vi "RCD TESTING.vi"(0 "Lock in Input":T1, 1 "error in (no error)":errorcluster, 2 "Deceleration":bool, 5 "RESET":bool, 6 "Accelaration":bool, 7 "B axis":i32, 8 "Stop":bool, 9 "A axis":i32, 10 "Comport":refnum<visa-resource-name>="COM4") -> (3 "A out":dbl, 4 "VISA resource name out":refnum<visa-resource-name>)   [LabVIEW 2020]
uses:
  <vilib>/Instr/_visa.llb/VISA Configure Serial Port (Instr).vi
  Dependencies/Holmarc/2 axis linear/GlobalValue.vi
  <vilib>/Utility/file.llb/Write Delimited Spreadsheet (DBL).vi
  Dependencies/Stanford Research 830/Stanford Research 830.lvlib
panel:
  out "Waveform Graph":sgl[](graph)
  in  "Maximum Time (10000 ms)":u32=10000
  in  "Continuous Storage (T: Enable)":bool=TRUE
  in  "Reset (True)":bool=TRUE
  in  "Sample Rate (0: 62.5 mHz)":u16(ring) items=["62.5 mHz", "125 mHz", "250 mHz", "500 mHz", "1 Hz", "2 Hz", "4 Hz", "8Hz", "16 Hz", "32 Hz", "64 Hz", "128 Hz", "256 Hz", "512 Hz", "Trigger "]
  out "error out 2":errorcluster
  out "B out":dbl
  # "COMPORT"
  # "To Move"
  # "Moved"
  # "Microns"
  # "Microns"
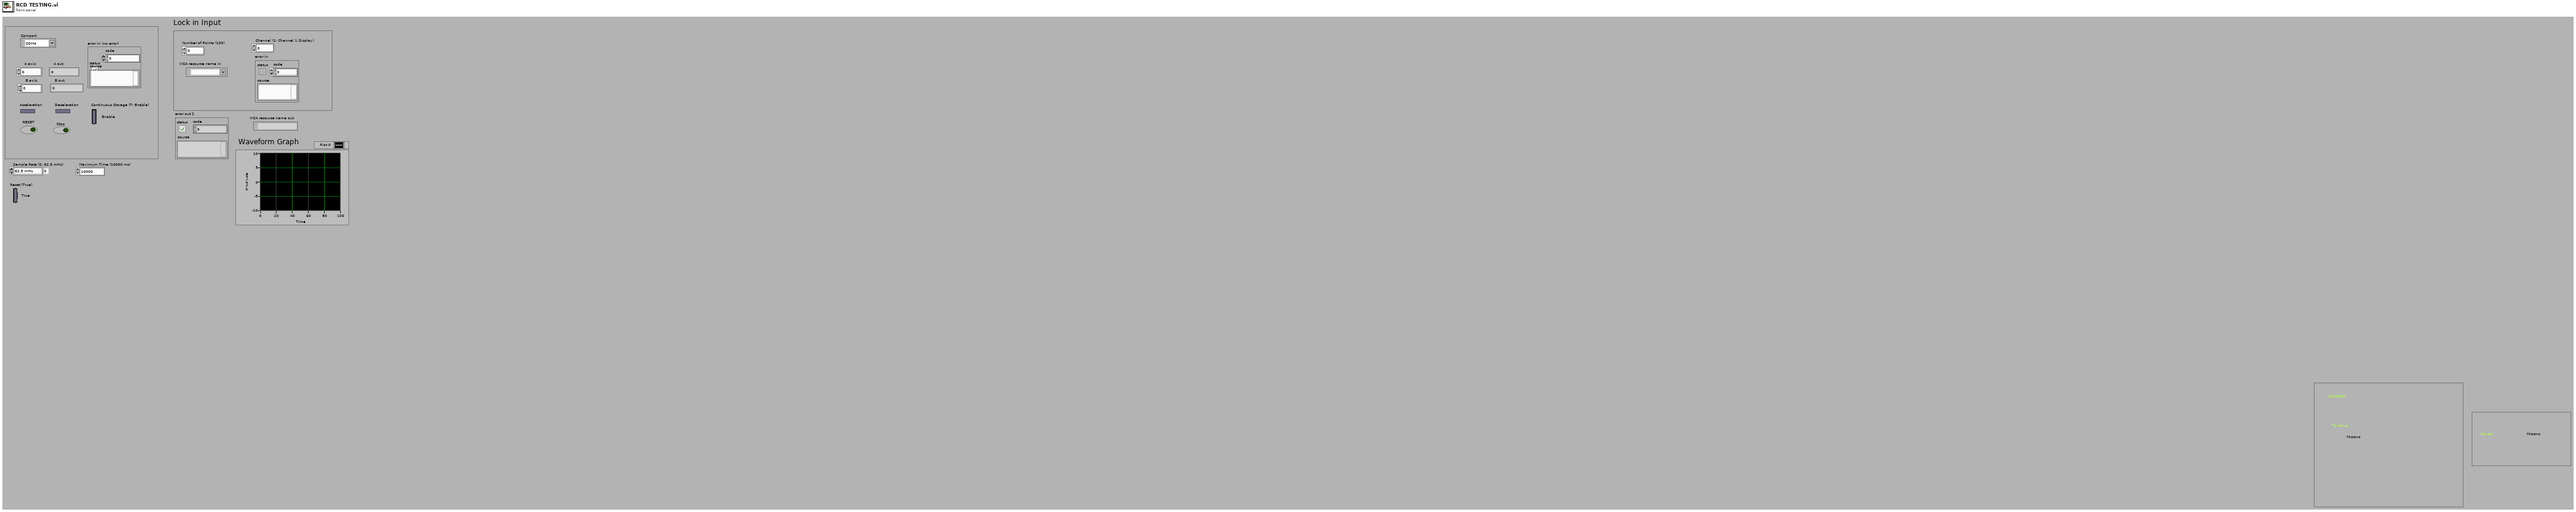
[diagram p1: front panel]
types:
  T1 = cluster{"Number of Points (100)":u32, "VISA resource name in":refnum<visa-resource-name>, "Channel (1: Channel 1 Display)":u16, "error in":errorcluster}
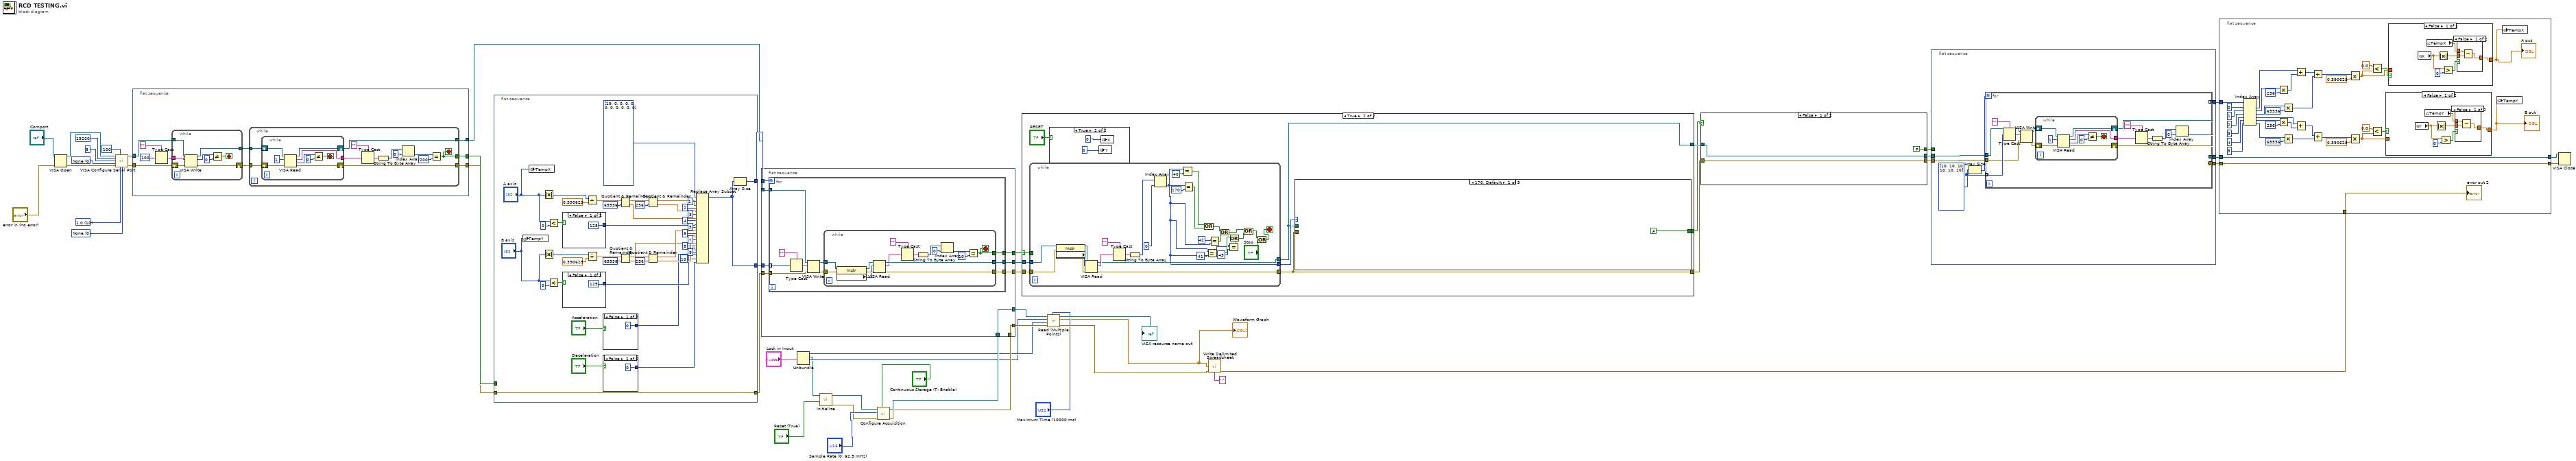
[diagram p0: block diagram]
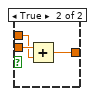
[diagram p2: hidden frame]
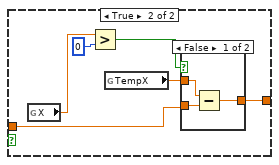
[diagram p3: hidden frame]
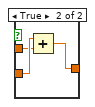
[diagram p4: hidden frame]
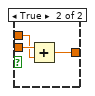
[diagram p5: hidden frame]
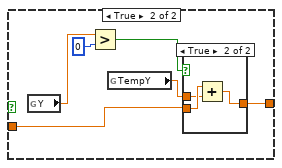
[diagram p6: hidden frame]
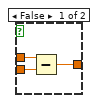
[diagram p7: hidden frame]
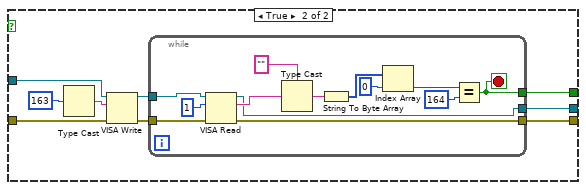
[diagram p8: hidden frame]
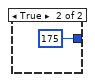
[diagram p9: hidden frame]
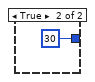
[diagram p10: hidden frame]
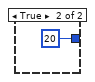
[diagram p11: hidden frame]
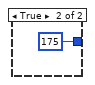
[diagram p12: hidden frame]
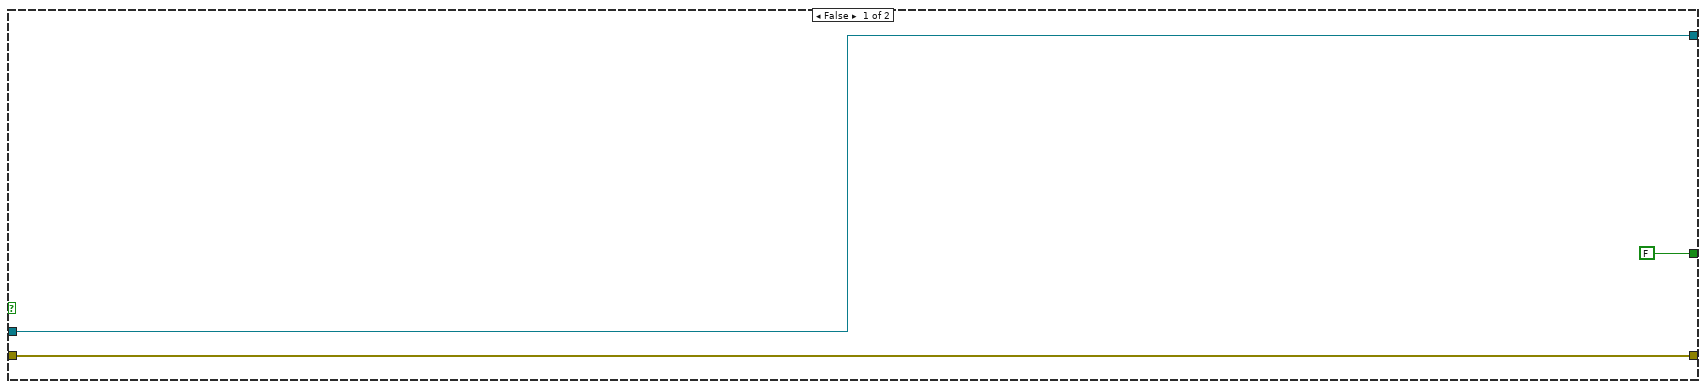
[diagram p13: hidden frame]
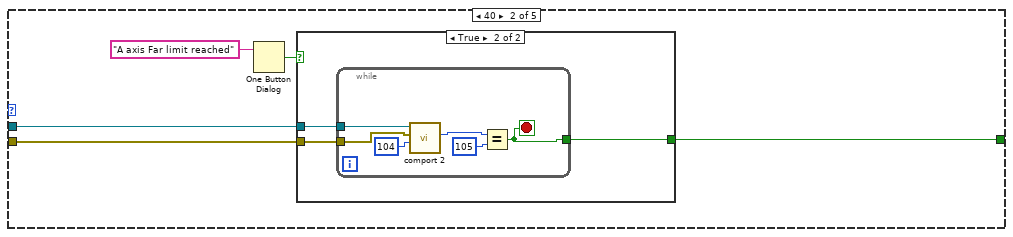
[diagram p15: hidden frame]
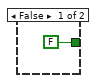
[diagram p16: hidden frame]
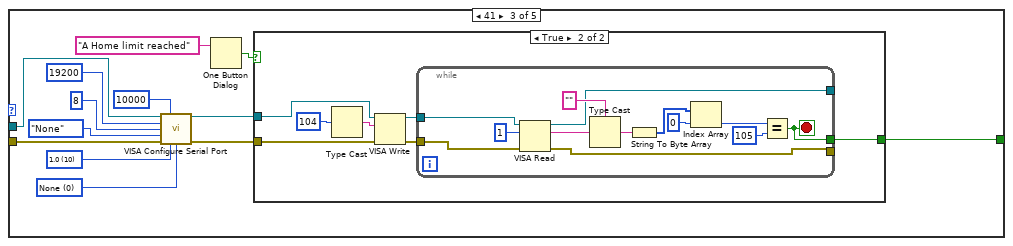
[diagram p17: hidden frame]
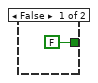
[diagram p18: hidden frame]
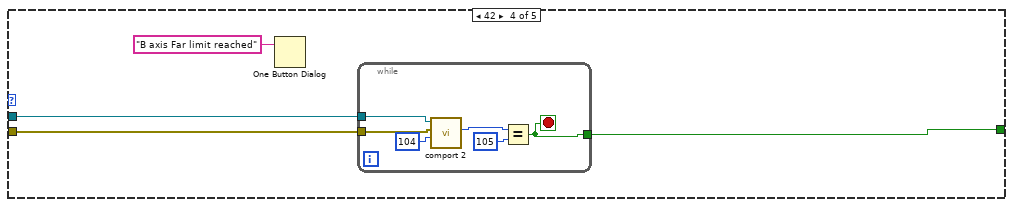
[diagram p19: hidden frame]
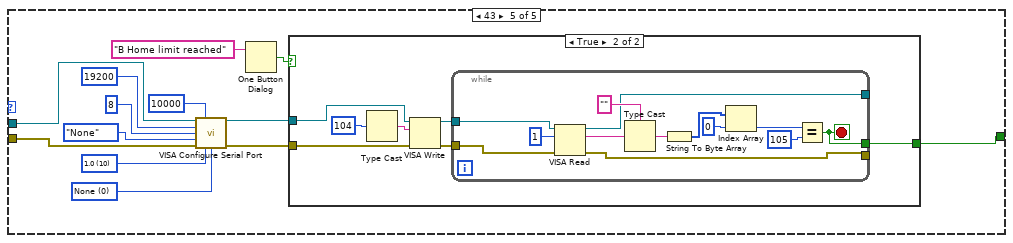
[diagram p20: hidden frame]
diagram:
  w46 = u16 0 items=["None"=0, "XON/XOFF"=1, "RTS/CTS"=2, "DTR/DSR"=4] ("flow control")
  w45 = u16 10 items=["1.0"=10, "1.5"=15, "2.0"=20] ("stop bits")
  w44 = u16 0 items=["None", "Odd", "Even", "Mark", "Space"] ("parity")
  n1 = VISA Open(error in (no error)="error in (no error)", VISA resource name="Comport") -> (VISA resource name=w49:refnum<visa-resource-name>, error out=w50:errorcluster)  [unwired: 3 in]
  n2 = call-poly "VISA Configure Serial Port"("VISA resource name"=w49, "timeout (10sec)"=u32 100, "baud rate (9600)"=u32 19200 ("baud rate"), "data bits (8)"=u16 8 ("data bits"), "parity (0:none)"=w44, "error in (no error)"=w50, "stop bits (10: 1 bit)"=w45, "flow control (0:none)"=w46) -> ("VISA resource name out"=w41:refnum<visa-resource-name>, "error out"=w40:errorcluster)  [unwired: 1 in, 5 out]
  n3 = flat-sequence {
    tunnel: w41 -> [w61]
    tunnel: w40 -> [w60]
    tunnel: [w59] -> w38
    tunnel: [w58] -> w25
    tunnel: [w52] -> w26
    frame #0 {
      n4 = Type Cast(type="", x=u8 100) -> (*(type *) &x=w56:string)
      n5 = while {
        tunnel: w56 -> [w69]
        shift-right: [w65] -> w53
        shift-left: w60 -> [w67]
        tunnel: w61 -> [w68]
        tunnel: [w66] -> w54
        stop <- w62 stop-if-true
        n6 = VISA Write(VISA resource name=w68, write buffer=w69, error in (no error)=w67) -> (VISA resource name out=w66:refnum<visa-resource-name>, return count=w64:u32, error out=w65:errorcluster)
        n7 = Not Equal?(x=w64, y=u32 0) -> (x != y?=w62:bool)
      }
      n8 = while {
        tunnel: w53 -> [w80]
        tunnel: [w78] -> w58
        tunnel: w54 -> [w81]
        tunnel: [w79] -> w59
        tunnel: [w73] -> w52
        stop <- w73 stop-if-true
        n9 = while {
          tunnel: [w85] -> w72
          shift-right: [w88] -> w79
          shift-left: w81 -> [w90]
          shift-right: [w87] -> w78
          shift-left: w80 -> [w89]
          stop <- w82 stop-if-true
          n10 = VISA Read(VISA resource name=w90, byte count=u32 1, error in (no error)=w89) -> (VISA resource name out=w88:refnum<visa-resource-name>, read buffer=w85:string, return count=w83:u32, error out=w87:errorcluster)
          n11 = Not Equal?(x=w83, y=u32 0) -> (x != y?=w82:bool)
        }
        n12 = Type Cast(type="", x=w72) -> (*(type *) &x=w70:string)
        n13 = String To Byte Array(string=w70) -> (unsigned byte array=w77:u8[])
        n14 = Index Array(array=w77, index=0) -> (element=w75:u8)
        n15 = Equal?(x=w75, y=u8 200) -> (x = y?=w73:bool)
      }
    }
  }
  n16 = flat-sequence {
    tunnel: [w129] -> w39
    tunnel: [w91] -> w37
    tunnel: w26 -> [_]
    tunnel: w25 -> [w126]
    tunnel: [w126] -> w24
    frame #0 {
      n17 = global write "GlobalValue.vi" "TempY"("B axis") -> ()
      n18 = global write "GlobalValue.vi" "TempX"("A axis") -> ()
      n19 = Absolute Value(x="A axis") -> (abs(x)=w130:i32)
      n20 = Absolute Value(x="B axis") -> (abs(x)=w118:i32)
      n21 = Less?(x="A axis", y=0) -> (x < y?=w132:bool)
      n22 = Less?(x="B axis", y=0) -> (x < y?=w113:bool)
      n23 = case shown="False" w132 {
        tunnel: [u16 125 u16 175] -> w104
        frame False {
        }
        frame True {
        }
      }
      n24 = case shown="False" w113 {
        tunnel: [u16 125 u16 175] -> w96
        frame False {
        }
        frame True {
        }
      }
      n25 = Divide(x=w130, y=0.390625) -> (x/y=w125:dbl)
      n26 = Divide(x=w118, y=0.390625) -> (x/y=w117:dbl)
      n27 = case shown="False" "Accelaration" {
        tunnel: [0 20] -> w94
        frame False {
        }
        frame True {
        }
      }
      n28 = case shown="False" "Deceleration" {
        tunnel: [0 30] -> w92
        frame False {
        }
        frame True {
        }
      }
      n29 = Quotient & Remainder(x=w125, y=65536) -> (x-y*floor(x/y)=w123:dbl, floor(x/y)=w107:dbl)
      n30 = Quotient & Remainder(x=w117, y=65536) -> (x-y*floor(x/y)=w115:dbl, floor(x/y)=w98:dbl)
      n31 = Quotient & Remainder(x=w123, y=256) -> (x-y*floor(x/y)=w110:dbl, floor(x/y)=w109:dbl)
      n32 = Quotient & Remainder(x=w115, y=256) -> (x-y*floor(x/y)=w102:dbl, floor(x/y)=w100:dbl)
      n33 = Replace Array Subset(array=u8[] [19, 0, 0, 0, 0, 0, 0, 0, 0, 0, 0], new element #1=w110, index #1=1 ("index"), new element #2=w109, index #2=2 ("index"), new element #3=w107, index #3=3 ("index"), new element #4=w104, index #4=4 ("index"), new element #5=w102, index #5=5 ("index"), new element #6=w100, index #6=6 ("index"), new element #7=w98, index #7=7 ("index"), new element #8=w96, index #8=8 ("index"), new element #9=w94, index #9=9 ("index"), new element #10=w92, index #10=10 ("index")) -> (w91:u8[])
      n34 = Array Size(array=w91) -> (size(s)=w129:i32)
    }
  }
  n35 = flat-sequence {
    tunnel: w39 -> [w151]
    tunnel: w38 -> [w150]
    tunnel: w24 -> [w149]
    tunnel: w37 -> [w148]
    tunnel: [w147] -> w36
    tunnel: [w146] -> w23
    tunnel: [w145] -> w35
    tunnel: [w143] -> w19
    tunnel: [w144] -> w18
    tunnel: w9 -> [w144]
    tunnel: w8 -> [w143]
    frame #0 {
      n36 = for {
        N: w151 -> [_]
        tunnel: [w156] -> w145
        tunnel: w150 -> [w160]
        tunnel: [w158] -> w147
        tunnel: w149 -> [w159]
        tunnel: [w157] -> w146
        tunnel: w148 -> [w153] mode=indexing
        n37 = Type Cast(type="", x=w153) -> (*(type *) &x=w152:string)
        n38 = VISA Write(VISA resource name=w160, write buffer=w152, error in (no error)=w159) -> (VISA resource name out=w155:refnum<visa-resource-name>, error out=w154:errorcluster)  [unwired: 1 out]
        n39 = while {
          tunnel: w154 -> [w165]
          tunnel: [w175] -> w157
          tunnel: w155 -> [w166]
          tunnel: [w176] -> w158
          tunnel: [w170] -> w156
          stop <- w170 stop-if-true
          n40 = property class="Instr"(reference=w166, error in=w165) -> (reference out=w164:refnum<visa-resource-name>, error out=w163:errorcluster, "Serial Settings:Number of Bytes at Serial Port"=w162:u32)
          n41 = VISA Read(VISA resource name=w164, byte count=w162, error in (no error)=w163) -> (VISA resource name out=w176:refnum<visa-resource-name>, read buffer=w169:string, error out=w175:errorcluster)  [unwired: 1 out]
          n42 = Type Cast(type="", x=w169) -> (*(type *) &x=w167:string)
          n43 = String To Byte Array(string=w167) -> (unsigned byte array=w174:u8[])
          n44 = Index Array(array=w174, index=0) -> (element=w172:u8)
          n45 = Equal?(x=w172, y=u8 10) -> (x = y?=w170:bool)
        }
      }
    }
  }
  n46 = Unbundle("Lock in Input") -> ("Number of Points (100)"=w5:u32, "VISA resource name in"=w3:refnum<visa-resource-name>, "Channel (1: Channel 1 Display)"=w4:u16)  [unwired: 1 out]
  n47 = call "Initialize.vi"("Reset (True)"="Reset (True)", "VISA resource name"=w3) -> ("error out"=w11:errorcluster, "VISA resource name out"=w12:refnum<visa-resource-name>)  [unwired: 8 in]
  n48 = call "Configure Acquisition.vi"("Continuous Storage (T: Enable)"="Continuous Storage (T: Enable)", "error in (no error)"=w11, "Sample Rate (0: 62.5 mHz)"="Sample Rate (0: 62.5 mHz)", "VISA resource name"=w12) -> ("error out"=w8:errorcluster, "VISA resource name out"=w9:refnum<visa-resource-name>)  [unwired: 6 in]
  n49 = case shown="True" w35 {
    selector: w35 -> [_ w180]
    tunnel: w36 -> [w179 w184]
    tunnel: w23 -> [w178 w186]
    tunnel: [w179 w183] -> w34
    tunnel: [w178 w182] -> w33
    tunnel: [FALSE w181] -> w20
    frame False {
    }
    frame True {
      n50 = while {
        tunnel: w186 -> [w202]
        tunnel: [w206] -> w183
        tunnel: [w208] -> w182
        tunnel: [w188] -> w185
        tunnel: w184 -> [w203]
        tunnel: w180 -> [_]
        stop <- w189 stop-if-true
        n51 = property class="Instr"(reference=w203, error in=w202) -> (reference out=w201:refnum<visa-resource-name>, error out=w200:errorcluster, "Serial Settings:Number of Bytes at Serial Port"=w199:u32)
        n52 = VISA Read(VISA resource name=w201, byte count=w199, error in (no error)=w200) -> (VISA resource name out=w206:refnum<visa-resource-name>, read buffer=w215:string, error out=w208:errorcluster)  [unwired: 1 out]
        n53 = Type Cast(type="", x=w215) -> (*(type *) &x=w216:string)
        n54 = String To Byte Array(string=w216) -> (unsigned byte array=w214:u8[])
        n55 = Index Array(array=w214, index=0) -> (element=w188:u8)
        n56 = Equal?(x=w188, y=u8 40) -> (x = y?=w205:bool)
        n57 = Equal?(x=w188, y=u8 170) -> (x = y?=w207:bool)
        n58 = Or(x=w205, y=w207) -> (x .or. y?=w196:bool)
        n59 = Equal?(x=w188, y=u8 41) -> (x = y?=w194:bool)
        n60 = Equal?(x=u8 42 ("y"), y=w188) -> (x = y?=w195:bool)
        n61 = Or(x=w196, y=w195) -> (x .or. y?=w204:bool)
        n62 = Equal?(x=w188, y=u8 43) -> (x = y?=w193:bool)
        n63 = Or(x=w194, y=w193) -> (x .or. y?=w192:bool)
        n64 = Or(x=w204, y=w192) -> (x .or. y?=w191:bool)
        n65 = Or(x=w191, y="Stop") -> (x .or. y?=w189:bool)
      }
      n66 = case shown="True" "RESET" {
        frame False {
        }
        frame True {
          n67 = global write "GlobalValue.vi" "Y"(0) -> ()
          n68 = global write "GlobalValue.vi" "X"(0) -> ()
        }
      }
      n69 = case shown="170, Default" w185 {
        tunnel: w183 -> [_ w221 w244 w271 w281]
        tunnel: w182 -> [_ w222 w241 w270 w280]
        tunnel: [FALSE w220 w245 w269 w279] -> w181
        frame 170, Default {
        }
        frame 40 {
          n70 = One Button Dialog(message="A axis Far limit reached") -> (true=w223:bool)  [unwired: 1 in]
          n71 = case shown="True" w223 {
            tunnel: w222 -> [_ w227]
            tunnel: w221 -> [_ w228]
            tunnel: [FALSE w226] -> w220
            frame False {
            }
            frame True {
              n72 = while {
                tunnel: w228 -> [w234]
                tunnel: w227 -> [w233]
                tunnel: [w229] -> w226
                stop <- w229 stop-if-true
                n73 = call "comport 2.vi"("x"=u8 104, "error in (no error)"=w233, "VISA resource name"=w234) -> ("Numeric"=w231:u8)  [unwired: 6 in, 2 out]
                n74 = Equal?(x=w231, y=u8 105) -> (x = y?=w229:bool)
              }
            }
          }
        }
        frame 41 {
          w236 = u16 0 items=["None", "XON/XOFF", "RTS/CTS", "XON/XOFF & RTS/CTS", "DTR/DSR", "XON/XOFF & DTR/DSR"] ("flow control (0:none)")
          w237 = u16 10 items=["1.0"=10, "1.5"=15, "2.0"=20] ("stop bits (10: 1 bit)")
          n75 = call-poly "VISA Configure Serial Port"("VISA resource name"=w244, "timeout (10sec)"=u32 10000, "baud rate (9600)"=u32 19200, "data bits (8)"=u16 8, "parity (0:none)"=enum16{"None", "Odd", "Even", "Mark", "Space"}."None", "error in (no error)"=w241, "stop bits (10: 1 bit)"=w237, "flow control (0:none)"=w236) -> ("VISA resource name out"=w243:refnum<visa-resource-name>, "error out"=w242:errorcluster)  [unwired: 6 in]
          n76 = One Button Dialog(message="A Home limit reached") -> (true=w246:bool)  [unwired: 1 in]
          n77 = case shown="True" w246 {
            tunnel: w243 -> [_ w252]
            tunnel: w242 -> [_ w251]
            tunnel: [FALSE w249] -> w245
            frame False {
            }
            frame True {
              n78 = Type Cast(x=104) -> (*(type *) &x=w255:string)  [unwired: 1 in]
              n79 = VISA Write(VISA resource name=w252, write buffer=w255, error in (no error)=w251) -> (VISA resource name out=w253:refnum<visa-resource-name>, error out=w254:errorcluster)  [unwired: 1 out]
              n80 = while {
                tunnel: w254 -> [w268]
                tunnel: [w258] -> _
                tunnel: w253 -> [w267]
                tunnel: [w257] -> _
                tunnel: [w256] -> w249
                stop <- w256 stop-if-true
                n81 = VISA Read(VISA resource name=w267, byte count=u32 1, error in (no error)=w268) -> (VISA resource name out=w257:refnum<visa-resource-name>, read buffer=w259:string, error out=w258:errorcluster)  [unwired: 1 out]
                n82 = Type Cast(type="", x=w259) -> (*(type *) &x=w260:string)
                n83 = String To Byte Array(string=w260) -> (unsigned byte array=w264:u8[])
                n84 = Index Array(array=w264, index=0) -> (element=w261:u8)
                n85 = Equal?(x=w261, y=u8 105) -> (x = y?=w256:bool)
              }
            }
          }
        }
        frame 42 {
          n86 = One Button Dialog(message="B axis Far limit reached") -> ()  [unwired: 1 in, 1 out]
          n87 = while {
            tunnel: [w275] -> w269
            tunnel: w271 -> [w274]
            tunnel: w270 -> [w273]
            stop <- w275 stop-if-true
            n88 = call "comport 2.vi"("x"=u8 104, "error in (no error)"=w273, "VISA resource name"=w274) -> ("Numeric"=w277:u8)  [unwired: 6 in, 2 out]
            n89 = Equal?(x=w277, y=u8 105) -> (x = y?=w275:bool)
          }
        }
        frame 43 {
          w283 = u16 0 items=["None", "XON/XOFF", "RTS/CTS", "XON/XOFF & RTS/CTS", "DTR/DSR", "XON/XOFF & DTR/DSR"] ("flow control (0:none)")
          w284 = u16 10 items=["1.0"=10, "1.5"=15, "2.0"=20] ("stop bits (10: 1 bit)")
          n90 = call-poly "VISA Configure Serial Port"("VISA resource name"=w281, "timeout (10sec)"=u32 10000, "baud rate (9600)"=u32 19200, "data bits (8)"=u16 8, "parity (0:none)"=enum16{"None", "Odd", "Even", "Mark", "Space"}."None", "error in (no error)"=w280, "stop bits (10: 1 bit)"=w284, "flow control (0:none)"=w283) -> ("VISA resource name out"=w289:refnum<visa-resource-name>, "error out"=w288:errorcluster)  [unwired: 6 in]
          n91 = One Button Dialog(message="B Home limit reached") -> (true=w290:bool)  [unwired: 1 in]
          n92 = case shown="True" w290 {
            tunnel: w289 -> [_ w296]
            tunnel: w288 -> [_ w295]
            tunnel: [FALSE w293] -> w279
            frame False {
            }
            frame True {
              n93 = Type Cast(x=104) -> (*(type *) &x=w299:string)  [unwired: 1 in]
              n94 = VISA Write(VISA resource name=w296, write buffer=w299, error in (no error)=w295) -> (VISA resource name out=w297:refnum<visa-resource-name>, error out=w298:errorcluster)  [unwired: 1 out]
              n95 = while {
                tunnel: w298 -> [w312]
                tunnel: [w302] -> _
                tunnel: w297 -> [w311]
                tunnel: [w301] -> _
                tunnel: [w300] -> w293
                stop <- w300 stop-if-true
                n96 = VISA Read(VISA resource name=w311, byte count=u32 1, error in (no error)=w312) -> (VISA resource name out=w301:refnum<visa-resource-name>, read buffer=w303:string, error out=w302:errorcluster)  [unwired: 1 out]
                n97 = Type Cast(type="", x=w303) -> (*(type *) &x=w304:string)
                n98 = String To Byte Array(string=w304) -> (unsigned byte array=w308:u8[])
                n99 = Index Array(array=w308, index=0) -> (element=w305:u8)
                n100 = Equal?(x=w305, y=u8 105) -> (x = y?=w300:bool)
              }
            }
          }
        }
      }
    }
  }
  n101 = call "Read (Multiple Points).vi"("Maximum Time (10000 ms)"="Maximum Time (10000 ms)", "error in (no error)"=w19, "Number of Points (100)"=w5, "Channel (1: Channel 1 Display)"=w4, "VISA resource name"=w18) -> ("error out"=w16:errorcluster, "Measurements"=w1:sgl[], "VISA resource name out"=→"VISA resource name out":refnum<visa-resource-name>)  [unwired: 4 in]
  "Waveform Graph" <- w1
  n102 = call-poly <vilib>:"Write Delimited Spreadsheet.vi"("1D data"=w1, "error in (no error)"=w16, "delimiter (\\t)"="." ("delimiter (\\t)")) -> ("error out"=w14:errorcluster)  [unwired: 11 in, 1 out]
  n103 = case shown="False" w20 {
    tunnel: w34 -> [w315 w321]
    tunnel: w33 -> [w314 w320]
    tunnel: [FALSE w319] -> w27
    tunnel: [w315 w317] -> w32
    tunnel: [w314 w318] -> w31
    frame False {
    }
    frame True {
      n104 = Type Cast(x=163) -> (*(type *) &x=w324:string)  [unwired: 1 in]
      n105 = VISA Write(VISA resource name=w321, write buffer=w324, error in (no error)=w320) -> (VISA resource name out=w322:refnum<visa-resource-name>, error out=w323:errorcluster)  [unwired: 1 out]
      n106 = while {
        tunnel: w323 -> [w337]
        tunnel: [w327] -> w318
        tunnel: w322 -> [w336]
        tunnel: [w326] -> w319
        tunnel: [w325] -> w317
        stop <- w326 stop-if-true
        n107 = VISA Read(VISA resource name=w336, byte count=u32 1, error in (no error)=w337) -> (VISA resource name out=w325:refnum<visa-resource-name>, read buffer=w328:string, error out=w327:errorcluster)  [unwired: 1 out]
        n108 = Type Cast(type="", x=w328) -> (*(type *) &x=w329:string)
        n109 = String To Byte Array(string=w329) -> (unsigned byte array=w333:u8[])
        n110 = Index Array(array=w333, index=0) -> (element=w330:u8)
        n111 = Equal?(x=w330, y=u8 164) -> (x = y?=w326:bool)
      }
    }
  }
  n112 = flat-sequence {
    tunnel: w31 -> [w343]
    tunnel: [w341] -> w29
    tunnel: [w342] -> w30
    tunnel: w32 -> [w340]
    tunnel: [w339] -> w28
    tunnel: w27 -> [_]
    frame #0 {
      w338 = u8[] [10, 10, 10, 10, 10, 10]
      n113 = Array Size(array=w338) -> (size(s)=w344:i32)
      n114 = for {
        N: w344 -> [_]
        tunnel: w343 -> [w347]
        tunnel: [w354] -> w342
        tunnel: w340 -> [w348]
        tunnel: [w353] -> w341
        tunnel: [w352] -> w339 mode=indexing
        tunnel: w338 -> [w349] mode=indexing
        n115 = Type Cast(type="", x=w349) -> (*(type *) &x=w350:string)
        n116 = VISA Write(VISA resource name=w348, write buffer=w350, error in (no error)=w347) -> (VISA resource name out=w346:refnum<visa-resource-name>, error out=w345:errorcluster)  [unwired: 1 out]
        n117 = while {
          tunnel: [w363] -> w357
          shift-right: [w366] -> w354
          shift-left: w346 -> [w368]
          shift-right: [w365] -> w353
          shift-left: w345 -> [w367]
          stop <- w360 stop-if-true
          n118 = VISA Read(VISA resource name=w368, byte count=u32 1, error in (no error)=w367) -> (VISA resource name out=w366:refnum<visa-resource-name>, read buffer=w363:string, return count=w361:u32, error out=w365:errorcluster)
          n119 = Not Equal?(x=w361, y=u32 0) -> (x != y?=w360:bool)
        }
        n120 = Type Cast(type="", x=w357) -> (*(type *) &x=w355:string)
        n121 = String To Byte Array(string=w355) -> (unsigned byte array=w359:u8[])
        n122 = Index Array(array=w359, index=0) -> (element=w352:u8)
      }
    }
  }
  n123 = flat-sequence {
    tunnel: w30 -> [w375]
    tunnel: w29 -> [w374]
    tunnel: w28 -> [w406]
    tunnel: [w375] -> w22
    tunnel: [w374] -> w21
    tunnel: w14 -> [w369]
    frame #0 {
      n124 = Index Array(array=w406, index #1=0 ("index"), index #2=1 ("index"), index #3=2 ("index"), index #4=3 ("index"), index #5=4 ("index"), index #6=5 ("index")) -> (element #1=w396:u8, element #2=w383:u8, element #3=w382:u8, element #4=w378:u8, element #5=w377:u8, element #6=w376:u8)
      n125 = Multiply(x=w383, y=u16 256) -> (x*y=w402:u16)
      n126 = Multiply(x=w377, y=u16 256) -> (x*y=w392:u16)
      n127 = Multiply(x=w382, y=u32 65536) -> (x*y=w401:u32)
      n128 = Multiply(x=w376, y=u32 65536) -> (x*y=w391:u32)
      n129 = Add(x=w396, y=w402) -> (x+y=w400:u16)
      n130 = Add(x=w378, y=w392) -> (x+y=w390:u16)
      n131 = Add(x=w400, y=w401) -> (x+y=w398:u32)
      n132 = Add(x=w390, y=w391) -> (x+y=w386:u32)
      n133 = Multiply(x=w398, y=0.390625) -> (x*y=w373:dbl)
      n134 = Multiply(x=w386, y=0.390625) -> (x*y=w387:dbl)
      n135 = Less?(x=0.0, y=w373) -> (x < y?=w370:bool)
      n136 = Less?(x=0.0, y=w387) -> (x < y?=w388:bool)
      n137 = case shown="False" w388 {
        tunnel: w387 -> [_ w443]
        tunnel: [w433 w445] -> w371
        frame False {
          n138 = global read "GlobalValue.vi" "Y"() -> (w432:dbl)
          n139 = global read "GlobalValue.vi" "TempY"() -> (w434:dbl)
          n140 = Absolute Value(x=w432) -> (abs(x)=w431:dbl)
          n141 = Greater?(x=w432, y=0) -> (0:w435:bool)
          n142 = case shown="False" w435 {
            tunnel: w431 -> [w438 w442]
            tunnel: w434 -> [w439 w441]
            tunnel: [w437 w440] -> w433
            frame False {
              n143 = Subtract(x=w439, y=w438) -> (x-y=w437:dbl)
            }
            frame True {
              n144 = Add(x=w442, y=w441) -> (x+y=w440:dbl)
            }
          }
        }
        frame True {
          n145 = global read "GlobalValue.vi" "Y"() -> (w444:dbl)
          n146 = Greater?(x=w444, y=0) -> (0:w447:bool)
          n147 = global read "GlobalValue.vi" "TempY"() -> (w446:dbl)
          n148 = case shown="True" w447 {
            tunnel: w443 -> [w450 w454]
            tunnel: w446 -> [w451 w453]
            tunnel: [w449 w452] -> w445
            frame False {
              n149 = Subtract(x=w451, y=w450) -> (x-y=w449:dbl)
            }
            frame True {
              n150 = Add(x=w454, y=w453) -> (x+y=w452:dbl)
            }
          }
        }
      }
      "B out" <- w371
      n151 = case shown="False" w370 {
        tunnel: w373 -> [_ w419]
        tunnel: [w409 w421] -> w372
        frame False {
          n152 = global read "GlobalValue.vi" "X"() -> (w408:dbl)
          n153 = global read "GlobalValue.vi" "TempX"() -> (w410:dbl)
          n154 = Absolute Value(x=w408) -> (abs(x)=w407:dbl)
          n155 = Greater?(x=w408, y=0) -> (0:w411:bool)
          n156 = case shown="False" w411 {
            tunnel: w407 -> [w414 w418]
            tunnel: w410 -> [w415 w417]
            tunnel: [w413 w416] -> w409
            frame False {
              n157 = Subtract(x=w415, y=w414) -> (x-y=w413:dbl)
            }
            frame True {
              n158 = Add(x=w418, y=w417) -> (x+y=w416:dbl)
            }
          }
        }
        frame True {
          n159 = global read "GlobalValue.vi" "X"() -> (w420:dbl)
          n160 = Greater?(x=w420, y=0) -> (0:w423:bool)
          n161 = global read "GlobalValue.vi" "TempX"() -> (w422:dbl)
          n162 = case shown="False" w423 {
            tunnel: w419 -> [w426 w430]
            tunnel: w422 -> [w427 w429]
            tunnel: [w425 w428] -> w421
            frame False {
              n163 = Subtract(x=w427, y=w426) -> (x-y=w425:dbl)
            }
            frame True {
              n164 = Add(x=w430, y=w429) -> (x+y=w428:dbl)
            }
          }
        }
      }
      "A out" <- w372
      n165 = global write "GlobalValue.vi" "TempY"(w371) -> ()
      n166 = global write "GlobalValue.vi" "TempX"(w372) -> ()
      "error out 2" <- w369
    }
  }
  n167 = VISA Close(VISA resource name=w22, error in (no error)=w21) -> ()  [unwired: 1 out]
